vi "Elapsed days.vi"(8 "error in":errorcluster, 10 "Second date":string="20/06/2008", 11 "First date":string="18/06/2007") -> (0 "error out":errorcluster, 3 "Elapsed days":dbl)   [LabVIEW 2013]
doc: "This VI outputs the number of elapsed days between two specified date strings. The VI converts the date strings to timestamps. It then uses those timestamps to calculate the number of elapsed days between the two dates."
panel:
  # "Select Help»Show Context Help and move the cursor \nover the VI icon to display help for this VI."
  # "Format: DD/MM/YY"
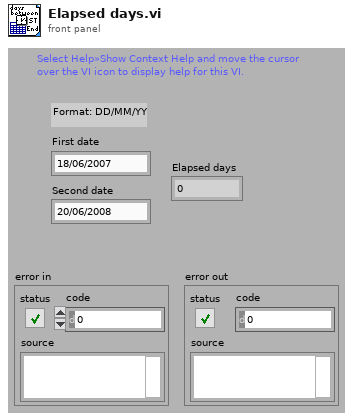
[diagram p1: front panel]
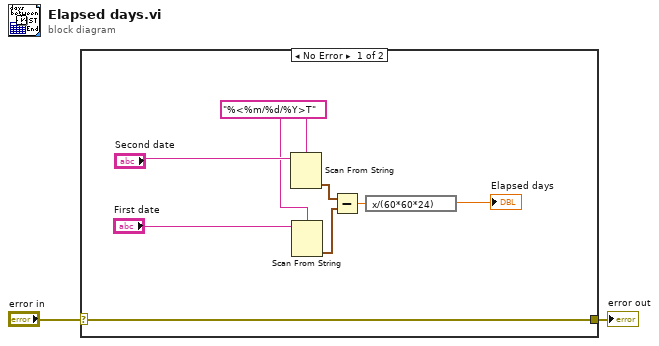
[diagram p0: block diagram]
diagram:
  n1 = case shown="No Error" "error in" {
    selector: "error in" -> [w3 w11]
    tunnel: [w3 w11] -> w1
    frame No Error {
      w8 = "%<%m/%d/%Y>T" ("format string")
      n2 = Scan From String(format string=w8, input string="Second date") -> (output 1=w7:timestamp)  [unwired: 3 in, 3 out]
      n3 = Scan From String(format string=w8, input string="First date") -> (output 1=w6:timestamp)  [unwired: 3 in, 3 out]
      n4 = Subtract(x=w7, y=w6) -> (x-y=w5:dbl)
      n5 = expression code="x/(60*60*24)"(w5) -> (→"Elapsed days":dbl)
    }
    frame Error {
    }
  }
  "error out" <- w1
